vi "Get_points_for_single_shot.vi"(0 "Control_interface in":refnum<class "Control_interface.lvclass">=refnum, 3 "error in (no error)":errorcluster) -> (7 "Control_interface out":refnum<class "Control_interface.lvclass">, 10 "error out":errorcluster)   [LabVIEW 2015, in "Control_interface.lvclass"]
uses:
  Control_interface.lvclass
panel:
  in  "Number of Points":dbl=8640.0 min=160.0 step=160.0
  in  "Press when finished":bool=TRUE
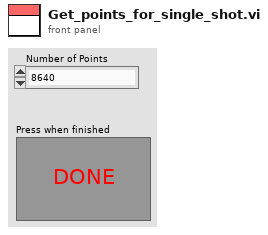
[diagram p1: front panel]
types:
  T1 = cluster{"Sample Rate":dbl, "Clock mode":enum16{"Internal", "External", "Reference"}, "Mode":u16, "Depth":dbl, "Segment Size":dbl, "Trigger Timeout":dbl, "Trigger Holdoff":dbl, "Trigger Delay":dbl}
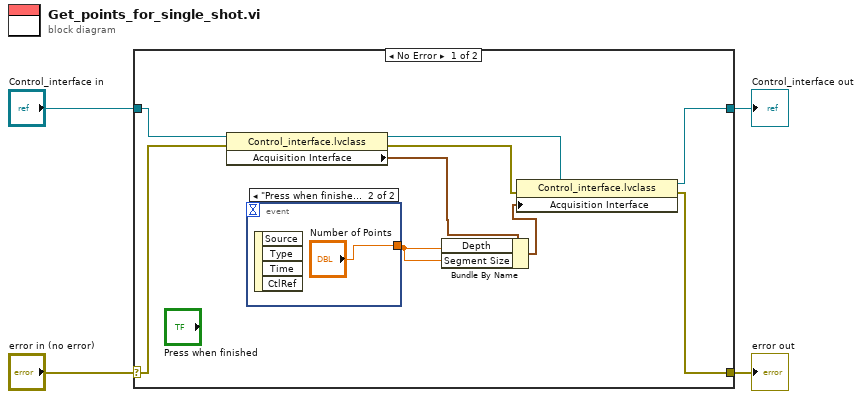
[diagram p0: block diagram]
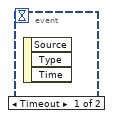
[diagram p2: hidden frame]
diagram:
  n1 = case shown="No Error" "error in (no error)" {
    selector: "error in (no error)" -> [w12 w16]
    tunnel: [w6 w16] -> w3
    tunnel: [w7 w15] -> w1
    tunnel: "Control_interface in" -> [w13 w15]
    frame No Error {
      n2 = property class="Control_interface.lvclass"(reference=w13, error in=w12) -> (reference out=w9:refnum<class "Control_interface.lvclass">, error out=w8:errorcluster, "Acquisition Interface"=w11:T1)
      n3 = event shown="[1] \"Press when finished\": Value Change" {
        selector: _ -> [_ _]
        dyn-events: _ -> [_ _]
        timeout: _ -> [_ _]
        tunnel: [_ "Number of Points"] -> w10
        event Timeout {
          n4 = event-data() -> ()  [unwired: 1 in, 3 out]
        }
        event "Press when finished": Value Change {
          n5 = event-data() -> ()  [unwired: 1 in, 4 out]
        }
      }
      n6 = Bundle By Name(cluster=w11, "Depth"=w10, "Segment Size"=w10) -> (w5:T1)
      n7 = property class="Control_interface.lvclass"(reference=w9, error in=w8, "Acquisition Interface"=w5) -> (reference out=w7:refnum<class "Control_interface.lvclass">, error out=w6:errorcluster)
    }
    frame Error {
    }
  }
  "error out" <- w3
  "Control_interface out" <- w1
